vi "PhotonCamera_GetVersion.vi"(11 "BaseNTName":string="/photonvision") -> (0 "error out":errorcluster, 3 "Version":string)   [LabVIEW 2019, in "PhotonVisionLib.lvlib"]
doc: "Returned photonvision version string\n\nInputs:\n - BaseNTName - string - Base Nework Table name. (Optional. Default: /photonvision )\n \nOutputs:\n - Version - string - Photonvision version string\n - Error Out -- Contains error information if a Network table ot other error occured."
uses:
  PhotonVisionLib.lvlib
  <vilib>/Rock Robotics/Network Tables/NT Read String.vi
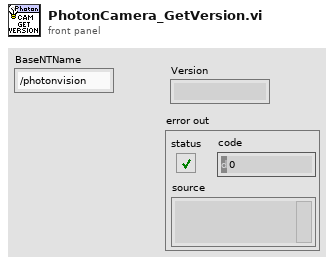
[diagram p1: front panel]
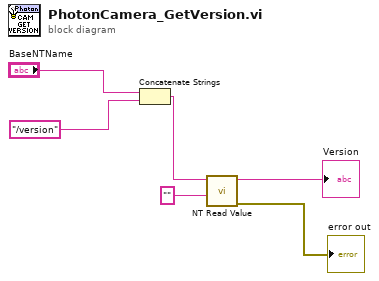
[diagram p0: block diagram]
diagram:
  n1 = Concatenate Strings("BaseNTName", "/version") -> (w1:string)
  n2 = call-poly <vilib>:"NT Read Value.vi"("default value"="", "name"=w1) -> ("error out"=→"error out":errorcluster, "value"=→"Version":string)  [unwired: 7 in, 1 out]
